vi "Analyze Core.vi"(8 "Error In":errorcluster, 10 "LHW-DataCollection in":refnum<class "LHW-DataCollection.lvclass">, 11 "LHW-Analysis-Actor in":refnum<class "LHW-Analysis-Actor.lvclass">) -> (0 "Error Out":errorcluster, 2 "LHW-DataCollection out":refnum<class "LHW-DataCollection.lvclass">, 3 "LHW-Analysis-Actor out":refnum<class "LHW-Analysis-Actor.lvclass">)   [LabVIEW 2016, in "LHW-Analysis.lvlib" / "LHW-Analysis-Actor.lvclass"]
doc: "Analyze received LHW-DataCollection, append result and update caller."
uses:
  LHW-Analysis-Actor.lvclass
  Classes/LHW-Data/LHW-DataCollection/LHW-DataCollection.lvclass
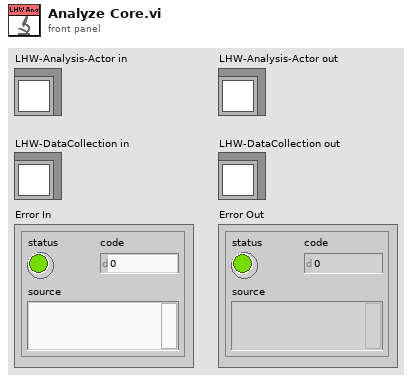
[diagram p1: front panel]
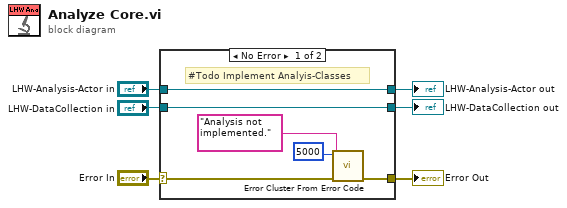
[diagram p0: block diagram]
diagram:
  n1 = case shown="No Error" "Error In" {
    selector: "Error In" -> [w8 w15]
    tunnel: [w7 w15] -> w5
    tunnel: [w12 w14] -> w3
    tunnel: "LHW-Analysis-Actor in" -> [w12 w14]
    tunnel: "LHW-DataCollection in" -> [w9 w13]
    tunnel: [w9 w13] -> w1
    frame No Error {
      # "#Todo Implement Analyis-Classes"
      n2 = call <vilib>:"Error Cluster From Error Code.vi"("error in (no error)"=w8, "error message (\"\")"="Analysis not implemented." ("error message (\"\")"), "error code (0)"=5000) -> ("error out"=w7:errorcluster)  [unwired: 6 in]
    }
    frame Error {
    }
  }
  "Error Out" <- w5
  "LHW-Analysis-Actor out" <- w3
  "LHW-DataCollection out" <- w1
